vi "Nest - Basic Read.vi"() -> ()   [LabVIEW 2013, in "LMH-Nest.lvlib"]
doc: "This example demonstrates how to read data from a Nest thermostat."
uses:
  vi.lib/MakerHub/Nest/LMH-Nest.lvlib
  vi.lib/MakerHub/Nest/Public/Get Temperature F.vi
  vi.lib/MakerHub/Nest/Public/Get Target Temperature F.vi
panel:
  out "Target Temp (F)":dbl
  out "Current Temp (F)":dbl
  in  "Nest Thermostat Name":string="Nest"
  in  "Password":string
  in  "Username (email)":string
  # "Nest Basic Read Example\n\nThis example demonstrates how to read data from a Nest thermostat.\n\n1. Enter your Username and Password in the Login section below.\n2. Enther the name you've assigned to your Nest.\n3. Click the Run Arrow.\n4. Notice the Current Temp and Target Temp are updated."
  # "Login"
  # "Nest Name"
  # "Temperature"
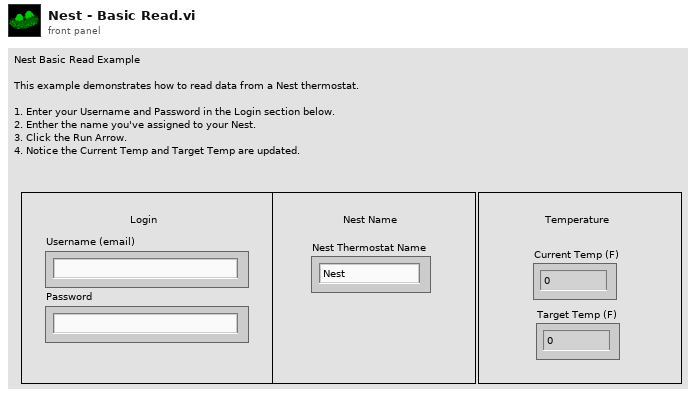
[diagram p1: front panel]
types:
  T1 = typedef "LMH-Nest.lvlib/Nest Config.ctl" = cluster{"Client Handle":T2, "Session Data":T3}
  T2 = typedef "LabVIEWHTTPClient.lvlib/ClientHandle.ctl" = refnum<k1>
  T3 = typedef "LMH-Nest.lvlib/Session Data.ctl" = cluster{"is_superuser":bool, "is_staff":bool, "urls":cluster{"transport_url":string, "rubyapi_url":string, "weather_url":string, "log_upload_url":string, "support_url":string}, "limits":cluster{"thermostats_per_structure":u32, "structures":u32, "thermostats":u32, "smoke_detectors":u32, "smoke_detectors_per_structure":u32}, "access_token":string, "userid":string, "expires_in":string, "email":string, "user":string, "language":string}
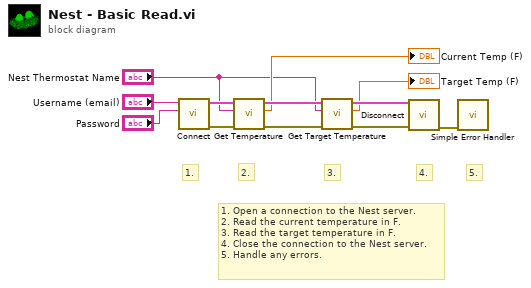
[diagram p0: block diagram]
diagram:
  # "1. Open a connection to the Nest server.\n2. Read the current temperature in F.\n3. Read the target temperature in F.\n4. Close the connection to the Nest server.\n5. Handle any errors."
  # "5."
  # "4."
  # "3."
  # "2."
  # "1."
  n1 = call "Connect.vi"("Password"="Password", "Username"="Username (email)") -> ("Error Out"=w7:errorcluster, "Nest Config"=w8:T1)  [unwired: 8 in]
  n2 = call-poly "Get Temperature.vi"("Error In"=w7, "Device Name"="Nest Thermostat Name", "Nest Config"=w8) -> ("Error Out"=w10:errorcluster, "Current Temp (F)"=→"Current Temp (F)":dbl, "Nest Config"=w9:T1)  [unwired: 6 in]
  n3 = call-poly "Get Target Temperature.vi"("Error In"=w10, "Device Name"="Nest Thermostat Name", "Nest Config"=w9) -> ("Error Out"=w5:errorcluster, "Target Temp (F)"=→"Target Temp (F)":dbl, "Nest Config"=w4:T1)  [unwired: 4 in, 2 out]
  n4 = call "Disconnect.vi"("Error In"=w5, "Nest Config"=w4) -> ("Error Out"=w2:errorcluster)  [unwired: 9 in]
  n5 = call <vilib>:"Simple Error Handler.vi"("error in (no error)"=w2) -> ()  [unwired: 4 in, 5 out]
